vi "Read Data.vi"(8 "error in (no error)":errorcluster, 11 "ScalarSignal in":refnum<class "ScalarSignal.lvclass">) -> (0 "error out":errorcluster, 2 "Data":dbl, 3 "ScalarSignal out":refnum<class "ScalarSignal.lvclass">)   [LabVIEW 2016, in "ScalarSignal.lvclass"]
uses:
  ScalarSignal.lvclass
  ScalarSignal.lvclass/ScalarSignal.ctl
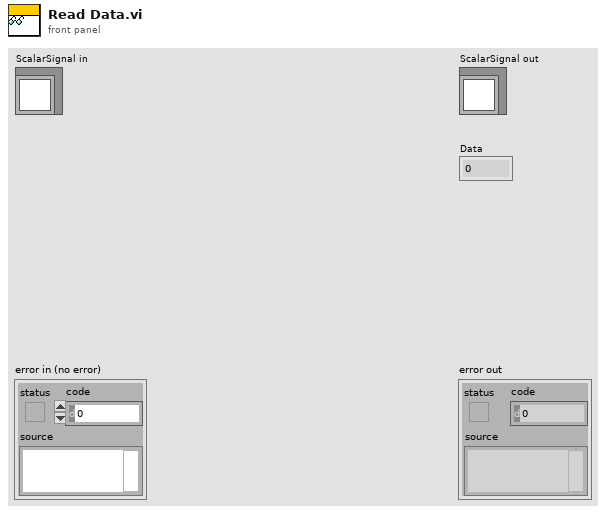
[diagram p1: front panel]
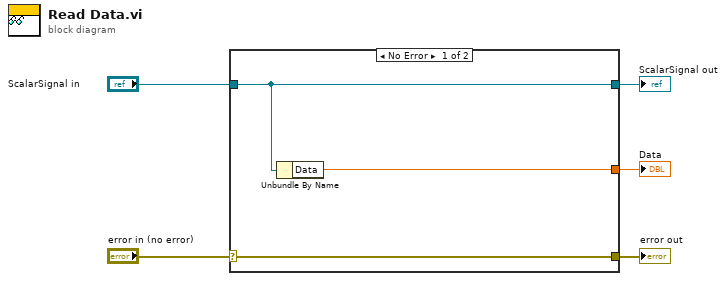
[diagram p0: block diagram]
diagram:
  n1 = case shown="No Error" "error in (no error)" {
    selector: "error in (no error)" -> [w8 w9]
    tunnel: [w8 w9] -> w4
    tunnel: [w7 w10] -> w2
    tunnel: "ScalarSignal in" -> [w7 w10]
    tunnel: [w6 _] -> w1
    frame No Error {
      n2 = Unbundle By Name(w7) -> ("Data"=w6:dbl)
    }
    frame Error {
    }
  }
  "error out" <- w4
  "ScalarSignal out" <- w2
  "Data" <- w1
